vi "Load Config File.vi"(8 "error in (no error)":errorcluster, 10 "Config File Path":path) -> (0 "error out":errorcluster, 3 "Json Instrument Configurations":string[](array[string]))   [LabVIEW 2020, in "JMETestSolutions.Instrument.lvlib" / "JMETestSolutions.Instrument.lvclass"]
doc: "This VI will Load a JSON Config File"
uses:
  JMETestSolutions.Instrument.lvclass
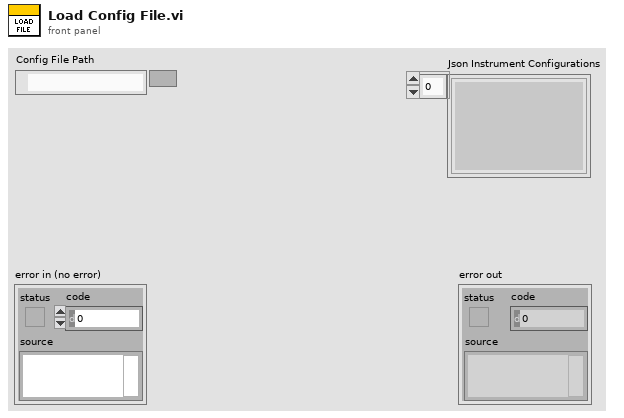
[diagram p1: front panel]
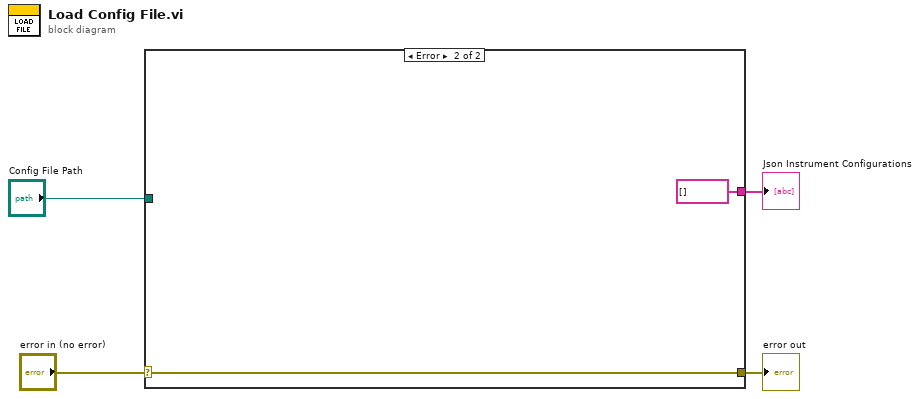
[diagram p0: block diagram]
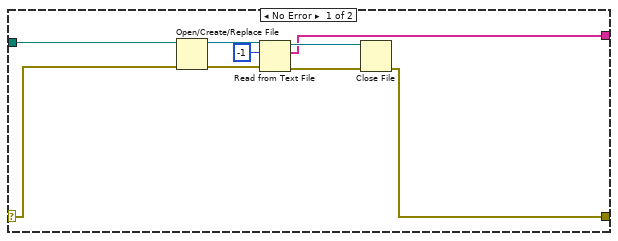
[diagram p2: hidden frame]
diagram:
  n1 = case shown="Error" "error in (no error)" {
    selector: "error in (no error)" -> [w12 w15]
    tunnel: [w7 w15] -> w3
    tunnel: "Config File Path" -> [w13 _]
    tunnel: [w5 string[] []] -> w1
    frame No Error {
      n2 = Open/Create/Replace File(file path (use dialog)=w13, error in=w12) -> (refnum out=w11:refnum<file>, error out=w10:errorcluster)  [unwired: 4 in, 1 out]
      n3 = Read from Text File(file (use dialog)=w11, count=-1, error in=w10) -> (refnum out=w9:refnum<file>, text=w5:string[], error out=w8:errorcluster)  [unwired: 1 in, 1 out]
      n4 = Close File(refnum=w9, error in=w8) -> (error out=w7:errorcluster)  [unwired: 1 out]
    }
    frame Error {
    }
  }
  "error out" <- w3
  "Json Instrument Configurations" <- w1
